vi "funcaoerro.vi"   [LabVIEW 2019]
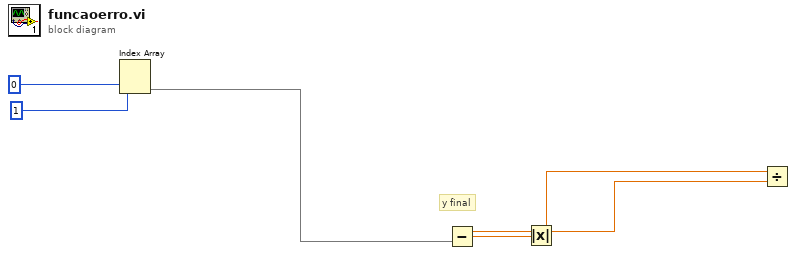
[diagram p0: block diagram]
diagram:
  # "y final"
  n1 = Index Array(index #1=0, index #2=1) -> (array=w6:dbl[], element #2=w1)  [unwired: 1 out]
  n2 = Subtract(y=w1) -> (x=w2:dbl, x-y=w4:dbl)
  n3 = Absolute Value(x=w4) -> (abs(x)=w3:dbl)
  n4 = Divide(x=w3, y=w2) -> ()  [unwired: 1 out]
